vi "create_filename.vi"(8 "Y":dbl, 9 "X":dbl, 10 "Index":i32, 11 "Base name":string) -> (3 "String 2":string)   [LabVIEW 2011]
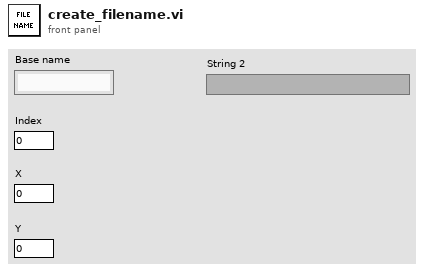
[diagram p1: front panel]
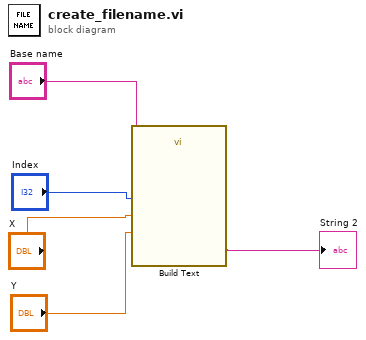
[diagram p0: block diagram]
diagram:
  n1 = call "Build Text"("Beginning Text"="Base name", "index"="Index", "x"="X", "y"="Y") -> ("Result"=→"String 2":string)  [unwired: 10 in, 1 out]
